vi "CoboltLaser_BasicWriteReadCheck.vi"(0 "ComPort":refnum<visa-resource-name>, 1 "Command":string, 3 "ExpectedResponseType":T1, 4 "ExpectedResponseMinimumLength":i32 min=0 step=1, 5 "ErrorMessage":string, 6 "GenerateError":bool, 7 "error in (no error)":errorcluster, 9 "Display Error message":bool) -> (20 "ComPortOut":refnum<visa-resource-name>, 21 "Response":string, 22 "ResponseOK":bool, 27 "error out":errorcluster)   [LabVIEW 2019]
doc: "Use this template to build a VI to use as a subVI."
uses:
  <userlib>/CoboltLaser/CoboltLaser_Controls/ExpectedResponseType.ctl
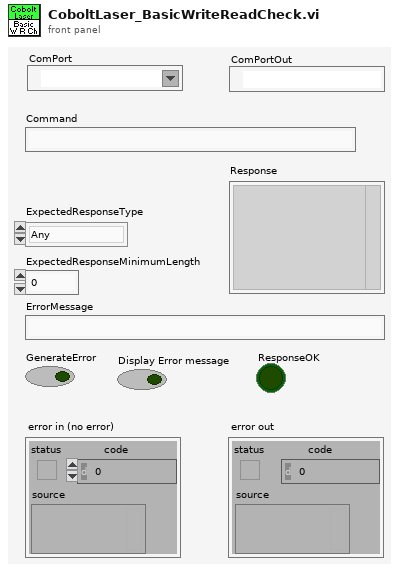
[diagram p1: front panel]
types:
  T1 = typedef "ExpectedResponseType.ctl" = enum16{"Any", "Digits Only", "Non-Digits Only"}
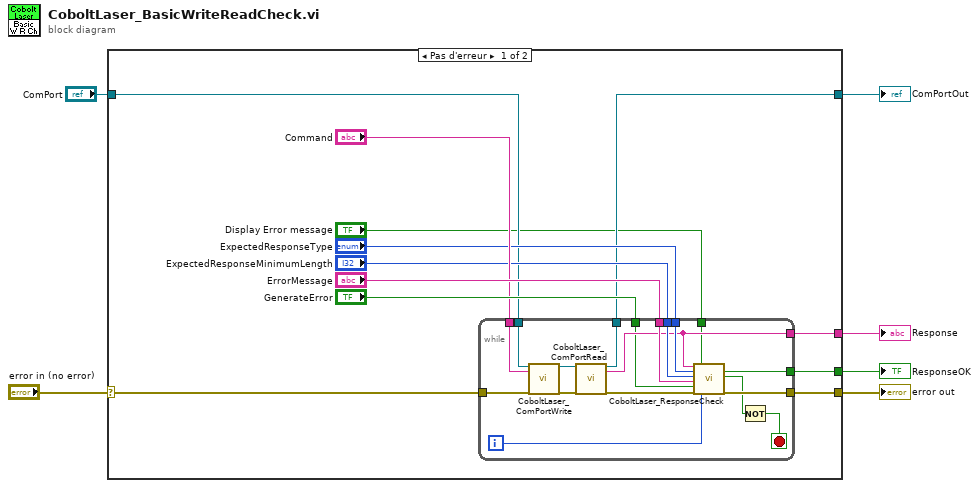
[diagram p0: block diagram]
diagram:
  n1 = case shown="Pas d'erreur" "error in (no error)" {
    selector: "error in (no error)" -> [w18 w38]
    tunnel: [w17 w38] -> w5
    tunnel: [w11 w37] -> w4
    tunnel: "ComPort" -> [w10 w37]
    tunnel: [w8 _] -> w2
    tunnel: [w7 _] -> w1
    frame No Error {
      n2 = while {
        tunnel: [w35] -> w11
        tunnel: [w34] -> w17
        tunnel: "GenerateError" -> [w23]
        tunnel: w10 -> [w33]
        tunnel: [w30] -> w8
        tunnel: "Command" -> [w29]
        tunnel: w18 -> [w28]
        tunnel: "ErrorMessage" -> [w27]
        tunnel: [w24] -> w7
        tunnel: "ExpectedResponseMinimumLength" -> [w25]
        tunnel: "ExpectedResponseType" -> [w26]
        tunnel: "Display Error message" -> [w19]
        i -> [w21]
        stop <- w22 stop-if-true
        n3 = call <userlib>:"CoboltLaser_ComPortWrite.vi"("ComPort"=w33, "Command"=w29, "error in (no error)"=w28) -> ("ComPortOut"=w32:refnum<visa-resource-name>, "error out"=w31:errorcluster)  [unwired: 15 in]
        n4 = call <userlib>:"CoboltLaser_ComPortRead.vi"("ComPort"=w32, "error in (no error)"=w31) -> ("ComPort Out"=w35:refnum<visa-resource-name>, "Response"=w24:string, "error out"=w36:errorcluster)  [unwired: 15 in]
        n5 = call <userlib>:"CoboltLaser_ResponseCheck.vi"("Response"=w24, "ExpectedResponseType"=w26, "ExpectedResponseMinimumLength"=w25, "ErrorMessage"=w27, "GenerateErrorIfFail"=w23, "ErrorIn"=w36, "Display Error message"=w19, "i"=w21) -> ("ResponseOK"=w30:bool, "Retry"=w20:bool, "ErrorOut"=w34:errorcluster)  [unwired: 9 in]
        n6 = Not(x=w20) -> (.not. x?=w22:bool)
      }
    }
    frame Error {
    }
  }
  "error out" <- w5
  "ComPortOut" <- w4
  "Response" <- w1
  "ResponseOK" <- w2
